vi "Init.vi"(8 "error in (no error)":errorcluster, 11 "Server":refnum<class "Server.lvclass">) -> (0 "error out":errorcluster, 3 "Arguments out":refnum<class "Arguments.lvclass">)   [LabVIEW 2020, in "HTTP Server.lvlib" / "Arguments.lvclass"]
uses:
  Arguments.lvclass
  Server/Server.lvclass
  Arguments.lvclass/Arguments.ctl
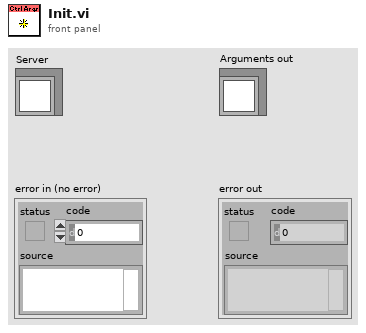
[diagram p1: front panel]
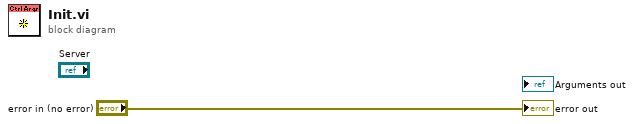
[diagram p0: block diagram]
diagram:
  "error out" <- "error in (no error)"
